vi "GetClassImplementationMethodNames.vi"(8 "error in (no error)":errorcluster, 11 "ClassReader in":refnum<class "ClassReader.lvclass">) -> (0 "error out":errorcluster, 2 "ImplementationMethodNames":string[](array[string]), 3 "ClassReader out":refnum<class "ClassReader.lvclass">)   [LabVIEW 2020, in "ClassReader.lvclass"]
uses:
  ClassReader.lvclass
  ClassReader.lvclass/ClassReader.ctl
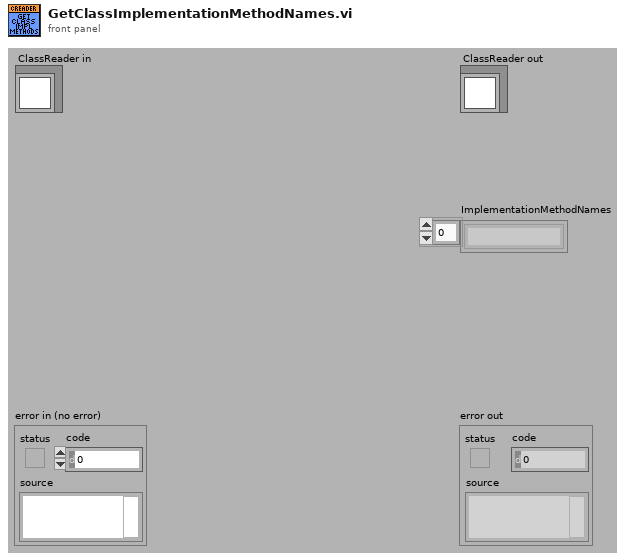
[diagram p1: front panel]
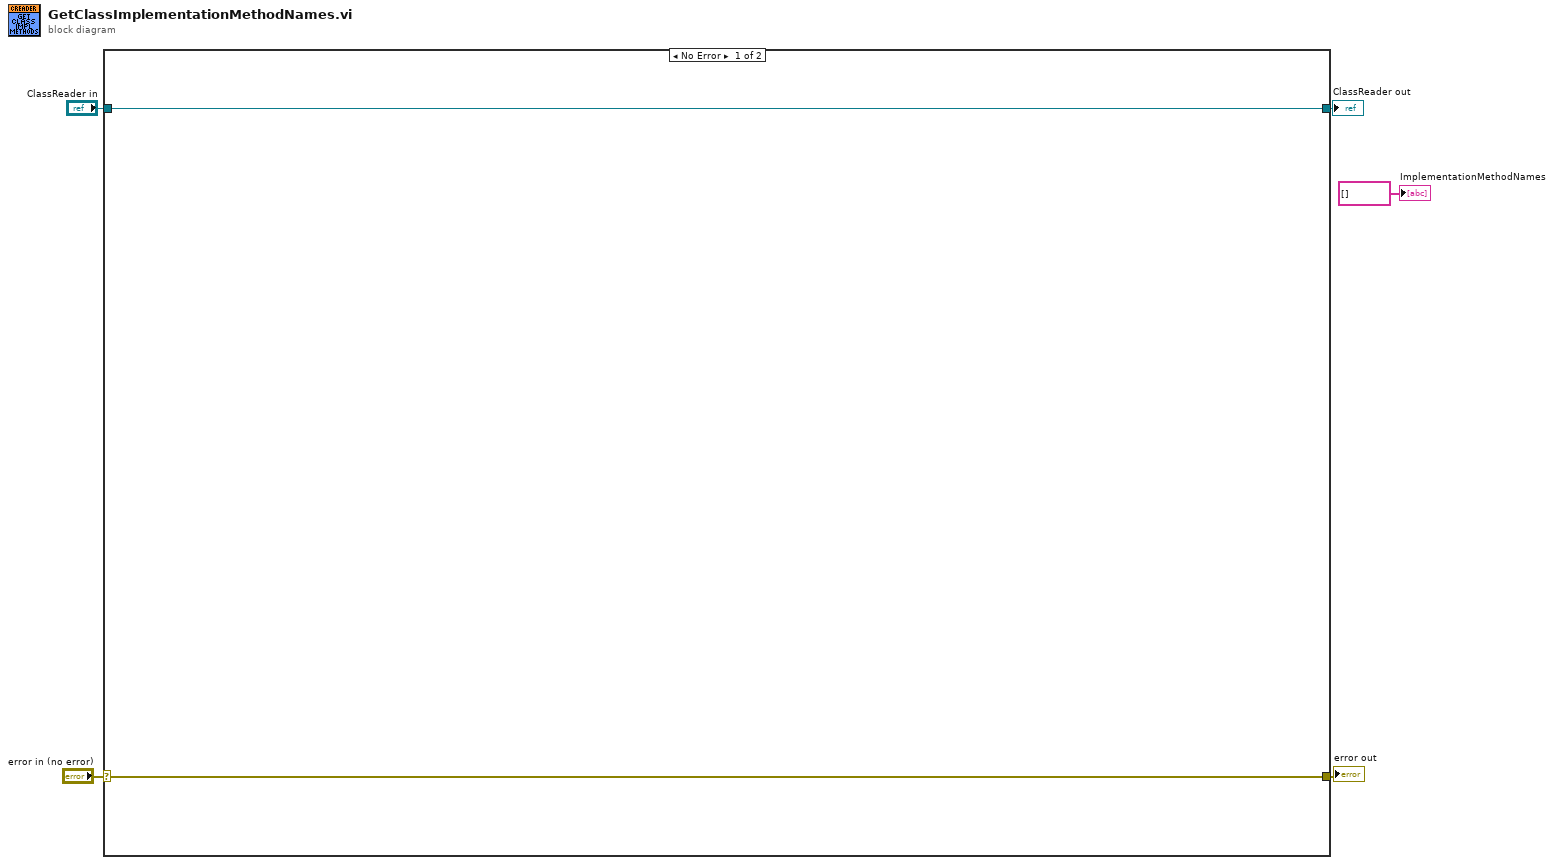
[diagram p0: block diagram]
diagram:
  n1 = case shown="No Error" "error in (no error)" {
    selector: "error in (no error)" -> [w6 w9]
    tunnel: [w6 w9] -> w4
    tunnel: [w7 w8] -> w2
    tunnel: "ClassReader in" -> [w7 w8]
    frame No Error {
    }
    frame Error {
    }
  }
  "error out" <- w4
  "ClassReader out" <- w2
  "ImplementationMethodNames" <- string[] [] ("ImplementationMethodNames")
